vi "Day 12 - Hill Climbing Algorithm.vi"() -> ()   [LabVIEW 2020, in "AoC 2022.lvlib"]
uses:
  AoC 2022.lvlib
  private/Paths.ctl
  private/Path.ctl
  private/Direction.ctl
  private/Route.ctl
panel:
  out "Routes out":T1[](array[typedef])
  out "Paths":T4
  out "Routes Visualisation":string[][][](array[string])
  out "String":string
  out "Path available ?":bool
  in  "Puzzle Input":string="Sabqponm\nabcryxxl\naccszExk\nacctuvwj\nabdefghi"
  out "Puzzle Part-2 Answer":string
  out "Puzzle Answer":string
  # "Press Ctrl+M & Enter the Puzzle Input and run the VI"
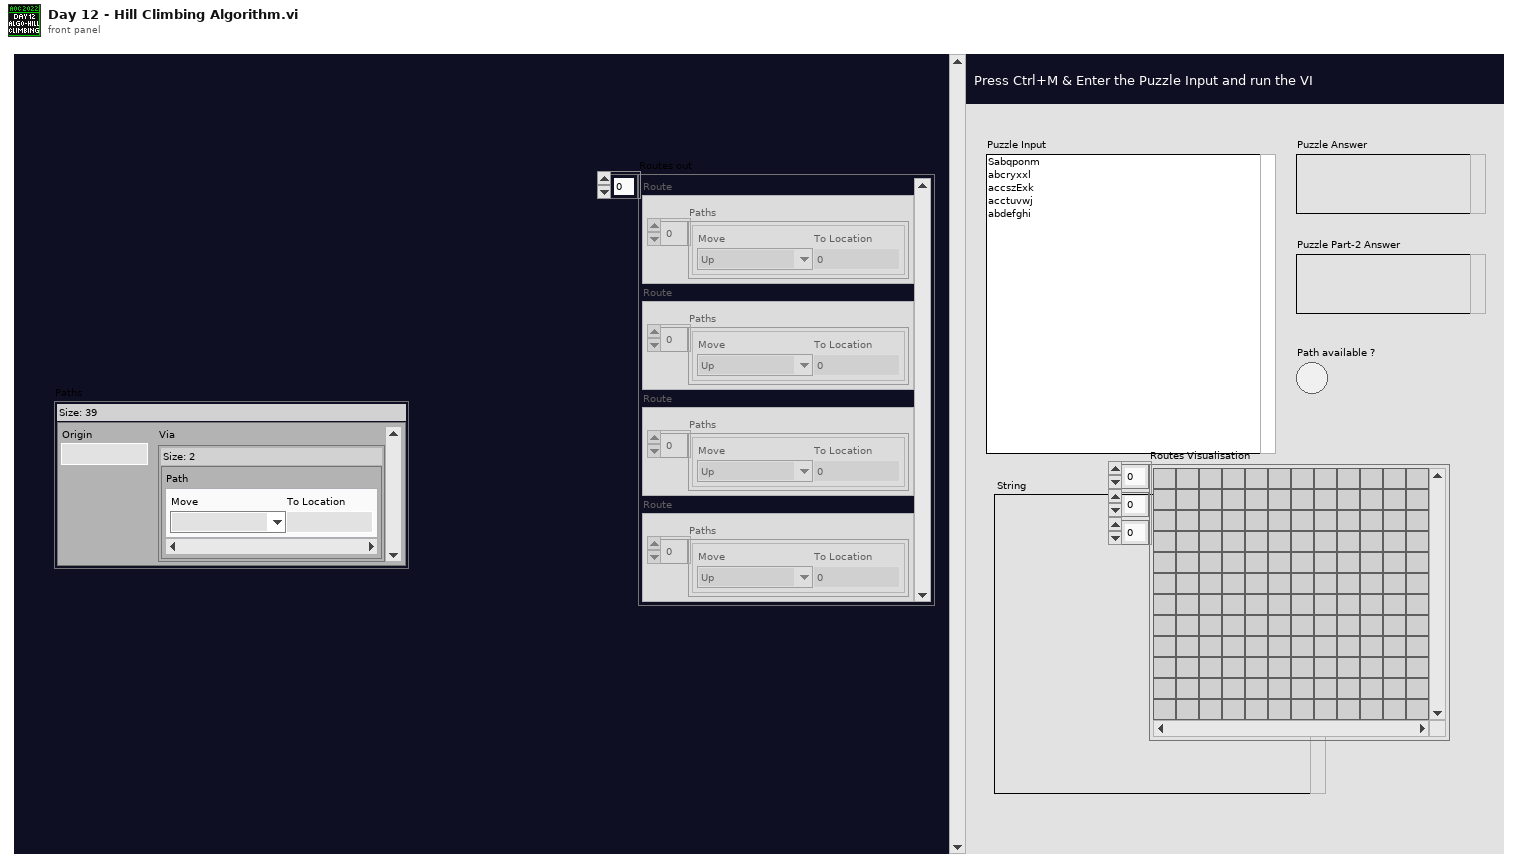
[diagram p1: front panel]
types:
  T1 = typedef "AoC 2022.lvlib/Route.ctl" = cluster{"Paths":T2[]}
  T2 = typedef "AoC 2022.lvlib/Path.ctl" = cluster{"Move":T3, "To Location":cdb}
  T3 = typedef "AoC 2022.lvlib/Direction.ctl" = enum16{"Up", "UpRight", "Right", "DownRight", "Down", "DownLeft", "Left", "UpLeft", "Stay"}
  T4 = typedef "AoC 2022.lvlib/Paths.ctl" = map{cdb, set{T2}}
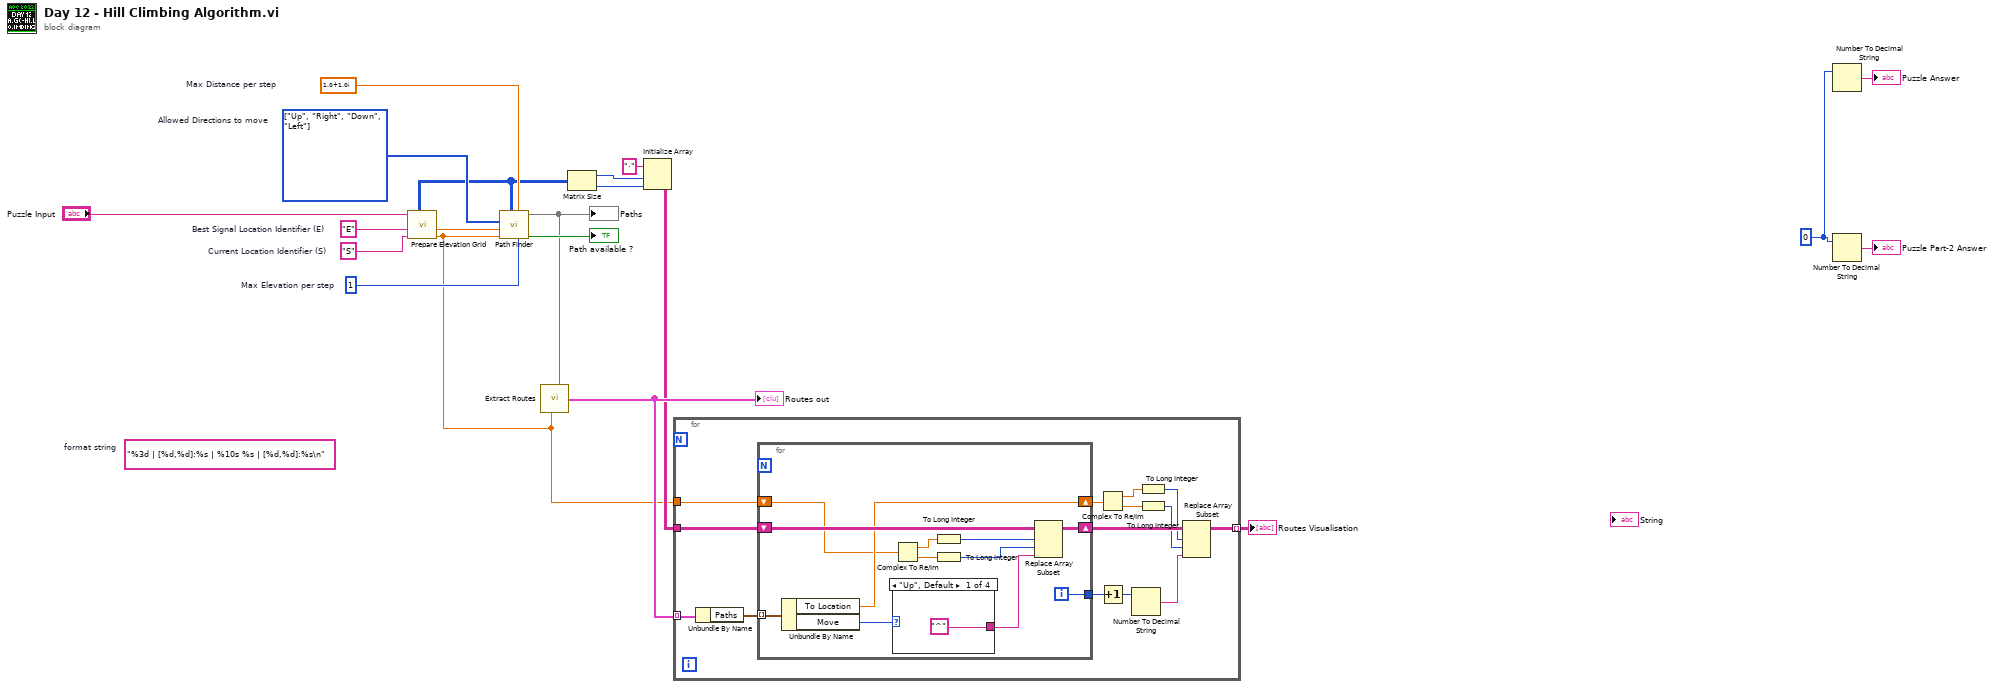
[diagram p0: block diagram]
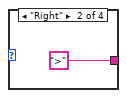
[diagram p2: hidden frame]
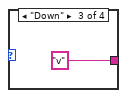
[diagram p3: hidden frame]
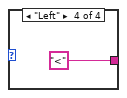
[diagram p4: hidden frame]
diagram:
  (unwired) "%3d | [%d,%d]:%s | %10s %s | [%d,%d]:%s\n"  # format string
  w13 = T3[] [enum."Up", enum."Right", enum."Down", enum."Left"] items=["Up", "UpRight", "Right", "DownRight", "Down", "DownLeft", "Left", "UpLeft", "Stay"]  # Allowed Directions to move
  w11 = "E"  # Best Signal Location Identifier (E)
  w12 = "S"  # Current Location Identifier (S)
  w16 = 1  # Max Elevation per step
  w15 = cdb 1.0+1.0i  # Max Distance per step
  w18 = 0
  n1 = call "Prepare Elevation Grid.vi"("Current Location Identifier (S)"=w12, "Best Signal Location Identifier (E)"=w11, "Plain Elevation Grid"="Puzzle Input") -> ("Current Location"=w1:cdb, "Best Signal Location"=w2:cdb, "Elevation Grid Numeric"=w8:i32[][])  [unwired: 3 in, 1 out]
  n2 = call "Path Finder.vi"("Allowed Directions to move"=w13, "Destination Location"=w2, "Current Location"=w1, "Elevation Grid Numeric"=w8, "Max Distance per step"=w15, "Max Elevation per step"=w16) -> ("Paths out"=w10:T4, "Path available ?"=→"Path available ?":bool)  [unwired: 3 in]
  "Paths" <- w10
  n3 = call "Extract Routes.vi"("From Location"=w1, "Paths in"=w10) -> ("Routes out"=w9:T1[])  [unwired: 1 in]
  "Routes out" <- w9
  n4 = Matrix Size(0:w8) -> (1:w7:i32, 2:w6:i32)
  n5 = Initialize Array("·", w7, w6) -> (w4:string[][])
  n6 = for {
    tunnel: w9 -> [w34] mode=indexing
    tunnel: w4 -> [w32]
    tunnel: [w29] -> w3 mode=indexing
    tunnel: w1 -> [w31]
    n7 = Unbundle By Name(w34) -> ("Paths"=w33:T2[])
    n8 = for {
      tunnel: w33 -> [w46] mode=indexing
      shift-right: [w44] -> w30
      shift-left: w32 -> [w45]
      shift-right: [w39] -> w26
      shift-left: w31 -> [w38]
      tunnel: [w35] -> w23
      i -> [w35]
      n9 = Unbundle By Name(w46) -> ("To Location"=w39:cdb, "Move"=w41:T3)
      n10 = case shown="\"Up\", Default" w41 {
        tunnel: ["^" ">" "v" "<"] -> w40
        frame "Up", Default {
        }
        frame "Right" {
        }
        frame "Down" {
        }
        frame "Left" {
        }
      }
      n11 = Complex To Re/Im(x + iy=w38) -> (x=w42:dbl, y=w43:dbl)
      n12 = To Long Integer(number=w42) -> (32bit integer=w37:i32)
      n13 = To Long Integer(number=w43) -> (32bit integer=w36:i32)
      n14 = Replace Array Subset(array=w45, new element=w40, index (row)=w37, index (col)=w36) -> (w44:string[][])
    }
    n15 = Complex To Re/Im(x + iy=w26) -> (x=w28:dbl, y=w27:dbl)
    n16 = Increment(x=w23) -> (x+1=w21:i32)
    n17 = Number To Decimal String(number=w21) -> (decimal integer string=w22:string)  [unwired: 1 in]
    n18 = To Long Integer(number=w28) -> (32bit integer=w25:i32)
    n19 = To Long Integer(number=w27) -> (32bit integer=w24:i32)
    n20 = Replace Array Subset(array=w30, new element=w22, index (row)=w25, index (col)=w24) -> (w29:string[][])
  }
  "Routes Visualisation" <- w3
  n21 = Number To Decimal String(number=w18) -> (decimal integer string=→"Puzzle Answer":string)  [unwired: 1 in]
  n22 = Number To Decimal String(number=w18) -> (decimal integer string=→"Puzzle Part-2 Answer":string)  [unwired: 1 in]
